vi "round_to_decimal.vi"(4 "Places after decimal point to round":sgl=1.0 min=0 step=1, 5 "Number to Round":dbl=4.999999969612645e-09) -> (2 "Rounded Number":dbl format="%#.10g")   [LabVIEW 2015]
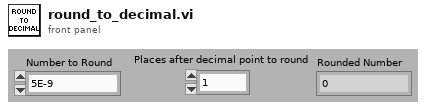
[diagram p1: front panel]
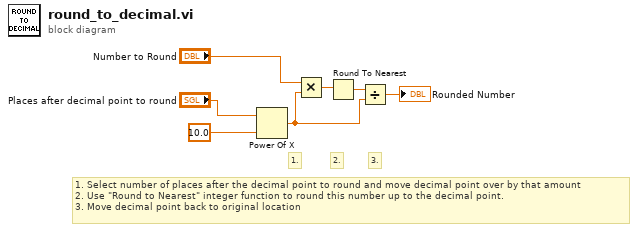
[diagram p0: block diagram]
diagram:
  # "3."
  # "1. Select number of places after the decimal point to round and move decimal point over by that amount\n2. Use \"Round to Nearest\" integer function to round this number up to the decimal point.\n3. Move decimal point back to original location"
  # "2."
  # "1."
  n1 = Power Of X(1:sgl 10.0 ("y"), 2:"Places after decimal point to round") -> (0:w2:sgl)
  n2 = Multiply(x="Number to Round", y=w2) -> (x*y=w6:dbl)
  n3 = Round To Nearest(number=w6) -> (nearest integer value=w5:dbl)
  n4 = Divide(x=w5, y=w2) -> (x/y=→"Rounded Number":dbl)
